vi "Global for ROS.vi"() -> ()   [LabVIEW 2015]
panel:
  in  "rosbridge server IP":string="192.168.1.117"
  in  "rosbridge port":u16=9090
  in  "Cluster":cluster{"Topic to write":string, "type":string}={"Topic to write"="rio", "type"="std_msgs/Int32MultiArray"}
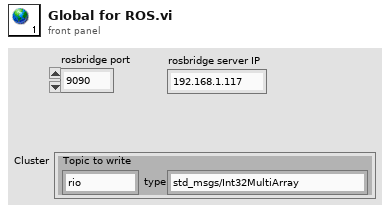
[diagram p1: front panel]
diagram:
